vi "Write output.vi"(8 "error in":errorcluster, 9 "data":u32[](array[numeric]), 11 "Run info":T1) -> (0 "error out":errorcluster, 3 "Run info out":T1)   [LabVIEW 2012]
uses:
  Run info.ctl
  <vilib>/DAQmx/write.llb/DAQmx Write (Digital 1D U32 1Chan NSamp).vi
  <vilib>/DAQmx/miscellaneous.llb/DAQmx Fill In Error Info.vi
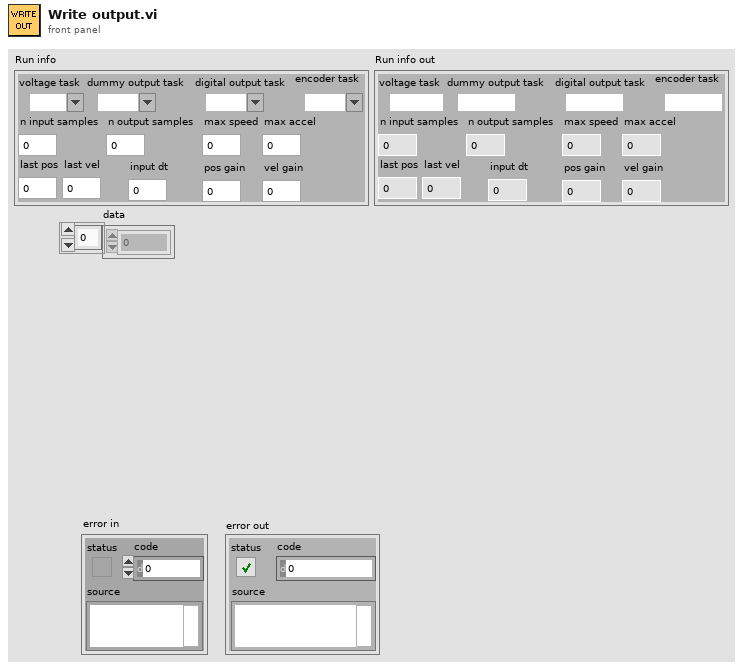
[diagram p1: front panel]
types:
  T1 = typedef "Run info.ctl" = cluster{"voltage task":refnum<k21>, "dummy output task":refnum<k21>, "digital output task":refnum<k21>, "encoder task":refnum<k21>, "n input samples":i32, "n output samples":i32, "max speed":dbl, "max accel":dbl, "last pos":dbl, "last vel":dbl, "pos gain":dbl, "vel gain":dbl, "input dt":dbl}
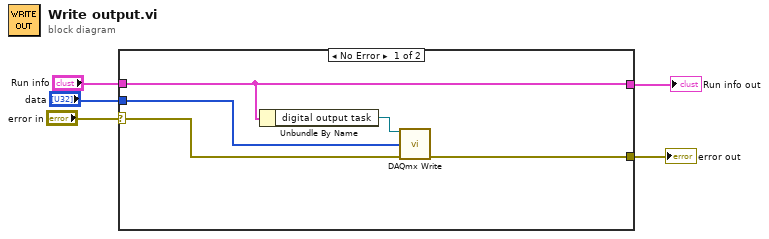
[diagram p0: block diagram]
diagram:
  n1 = case shown="No Error" "error in" {
    selector: "error in" -> [w6 w11]
    tunnel: "Run info" -> [w8 w12]
    tunnel: [w9 w11] -> w3
    tunnel: [w8 w12] -> w2
    tunnel: "data" -> [w7 _]
    frame No Error {
      n2 = Unbundle By Name(w8) -> ("digital output task"=w10:refnum<k21>)
      n3 = call-poly <vilib>:"DAQmx Write.vi"("task/channels in"=w10, "data"=w7, "error in"=w6) -> ("error out"=w9:errorcluster)  [unwired: 10 in, 2 out]
    }
    frame Error {
    }
  }
  "Run info out" <- w2
  "error out" <- w3
